vi "Close.vi"(8 "error in (no error)":errorcluster, 11 "TCatAdsNet in":refnum<class "AdsNET.lvclass">) -> (0 "error out":errorcluster)   [LabVIEW 2016, in "TCatAdsNet.lvlib" / "AdsNET.lvclass"]
doc: "Close ADS connection to server."
uses:
  AdsNET.lvclass
  AdsNET.lvclass/AdsNET.ctl
  C:/Users/Maurizio/Projects/twincat-lv-ads-library/TCatAdsNet Library/TwinCAT.Ads.dll
  TwinCAT.Ads.dll
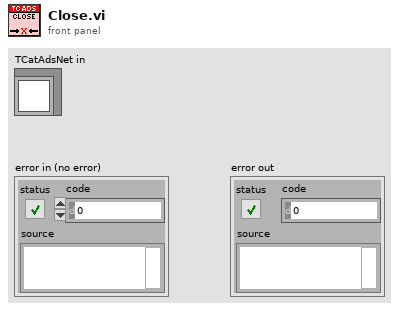
[diagram p1: front panel]
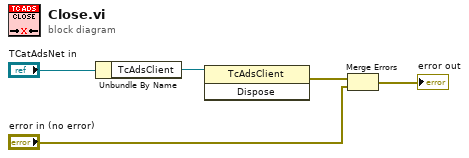
[diagram p0: block diagram]
diagram:
  n1 = Unbundle By Name("TCatAdsNet in") -> ("TcAdsClient"=w4:refnum<k24>)
  n2 = invoke class="TcAdsClient" method="Dispose"(reference=w4) -> (error out=w3:errorcluster)  [unwired: 2 in, 2 out]
  n3 = Merge Errors(w3, "error in (no error)") -> (→"error out":errorcluster)
